vi "JSONTimeToLVTime.vi"(11 "JSON time stamp":string) -> (3 "LV time stamp":timestamp)   [LabVIEW 2020, in "StashRoyale.lvclass"]
uses:
  StashRoyale.lvclass
  <vilib>/Utility/miscctls.llb/LVDateTimeRec.ctl
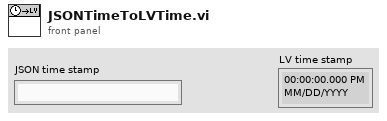
[diagram p1: front panel]
types:
  T1 = typedef "LVDateTimeRec.ctl" = cluster{"fractional second":dbl, "second":i32, "minute":i32, "hour":i32, "day of month":i32, "month":i32, "year":i32, "day of week":i32, "day of year":i32, "DST":i32}
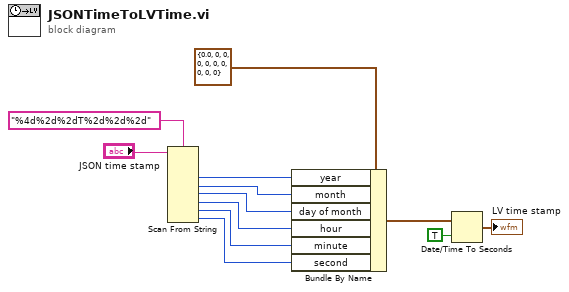
[diagram p0: block diagram]
diagram:
  n1 = Scan From String(format string="%4d%2d%2dT%2d%2d%2d", input string="JSON time stamp") -> (output 1=w9:i32, output 2=w8:i32, output 3=w7:i32, output 4=w6:i32, output 5=w5:i32, output 6=w4:i32)  [unwired: 8 in, 3 out]
  n2 = Bundle By Name(cluster=T1 {"fractional second"=0.0, "second"=0, "minute"=0, "hour"=0, "day of month"=0, "month"=0, "year"=0, "day of week"=0, "day of year"=0, "DST"=0} ("date time rec"), "year"=w9, "month"=w8, "day of month"=w7, "hour"=w6, "minute"=w5, "second"=w4) -> (w3:T1)
  n3 = Date/Time To Seconds(1:TRUE ("is UTC (F)"), 2:w3) -> (0:→"LV time stamp":timestamp)
